vi "Protocol Read to CRLF.vi"(8 "error in":errorcluster, 9 "timeout":i32=10000, 10 "bytes to read":i32, 11 "protocol layer in":refnum<class "Serial Slave.lvclass">) -> (0 "error out":errorcluster, 1 "timed out?":bool, 2 "data":u8[](array[numeric]), 3 "protocol layer out":refnum<class "Serial Slave.lvclass">)   [LabVIEW 2013, in "Serial Slave.lvclass"]
doc: "This provides an interface for reading from a network bus."
uses:
  Serial Slave.lvclass
  Serial Slave.lvclass/Serial Slave.ctl
  Serial Shared Components/Serial Shared Components.lvlib
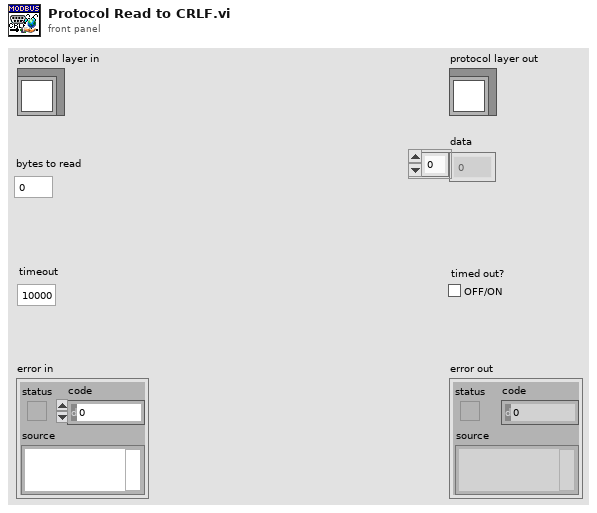
[diagram p1: front panel]
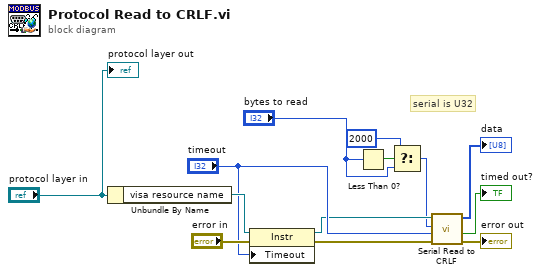
[diagram p0: block diagram]
diagram:
  # "serial is U32"
  n1 = Unbundle By Name("protocol layer in") -> ("visa resource name"=w7:refnum<visa-resource-name>)
  n2 = property class="Instr"(reference=w7, error in="error in", "Timeout"="timeout") -> (reference out=w5:refnum<visa-resource-name>, error out=w9:errorcluster)
  n3 = Less Than 0?(x="bytes to read") -> (x < 0?=w4:bool)
  n4 = Select(t=u32 2000, s=w4, f="bytes to read") -> (s? t:f=w2:u32)
  n5 = call "Serial Read to CRLF.vi"("error in"=w9, "timeout (ms)"="timeout", "bytes to read"=w2, "Visa Resource"=w5) -> ("error out"=→"error out":errorcluster, "timed out?"=→"timed out?":bool, "data"=→"data":u8[])  [unwired: 5 in]
  "protocol layer out" <- "protocol layer in"
